vi "Missing APU Value.vi"(10 "Num In":dbl, 11 "String In":string) -> (1 "Missing Value?":bool, 2 "Num Out":dbl, 3 "String Out":string)   [LabVIEW 2018]
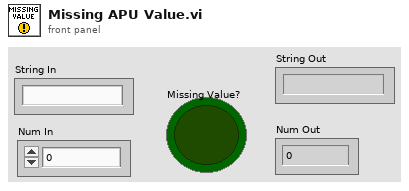
[diagram p1: front panel]
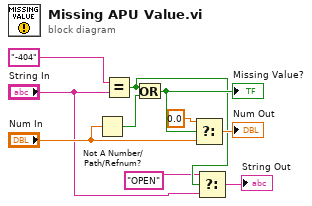
[diagram p0: block diagram]
diagram:
  n1 = Not A Number/Path/Refnum?(number/path/refnum="Num In") -> (NaN/Path/Refnum?=w9:bool)
  n2 = Equal?(x="-404", y="String In") -> (x = y?=w4:bool)
  n3 = Or(x=w4, y=w9) -> (x .or. y?=w8:bool)
  "Missing Value?" <- w8
  n4 = Select(t=0.0, s=w8, f="Num In") -> (s? t:f=→"Num Out":dbl)
  n5 = Select(t="OPEN", s=w4, f="String In") -> (s? t:f=→"String Out":string)
